vi "_fgv_attributes.vi"(6 "Attributes (empty)":T1[](array[typedef]) {"Flags" format="%08b"; "Access" items=["Read Only", "Write Only", "Read/Write"]; "Data Type" items=["Integer 32", "Double", "String", "Boolean", "None", "Integer 64", "RawString"]}, 7 "Operation":T5=enum."Get Attribute", 8 "error in":errorcluster caption="error in (no error)", 10 "Attribute ID in":string, 11 "VISA resource name":refnum<visa-resource-name>) -> (0 "error out":errorcluster, 1 "Count Out":i32, 2 "Attribute out":T2={"Identifier"="", "Descriptive Name"="", "Data Type"=enum."Integer 32", "Command"="", "Access"=enum."Read/Write", "Range Table"="", "Read Callback"="", "Write Callback"="", "Supported Models"="", "Instrument Options"="", "Index"=0, "OPC Wait"=FALSE, "No Status Check"=FALSE, "Cache Only"=FALSE}, 3 "VISA resource name out":refnum<visa-resource-name>)   [LabVIEW 2022 SP3, in "hmp4000_rsidr_core.lvlib"]
uses:
  hmp4000_rsidr_core.lvlib
  _type_Operation_Fgv_Attributes.ctl
  type_Attribute.ctl
  type_Attribute_Data_Type.ctl
  type_ReadWriteAccess.ctl
  type_Input_Format_Attribute.ctl
  type_Error_Codes.ctl
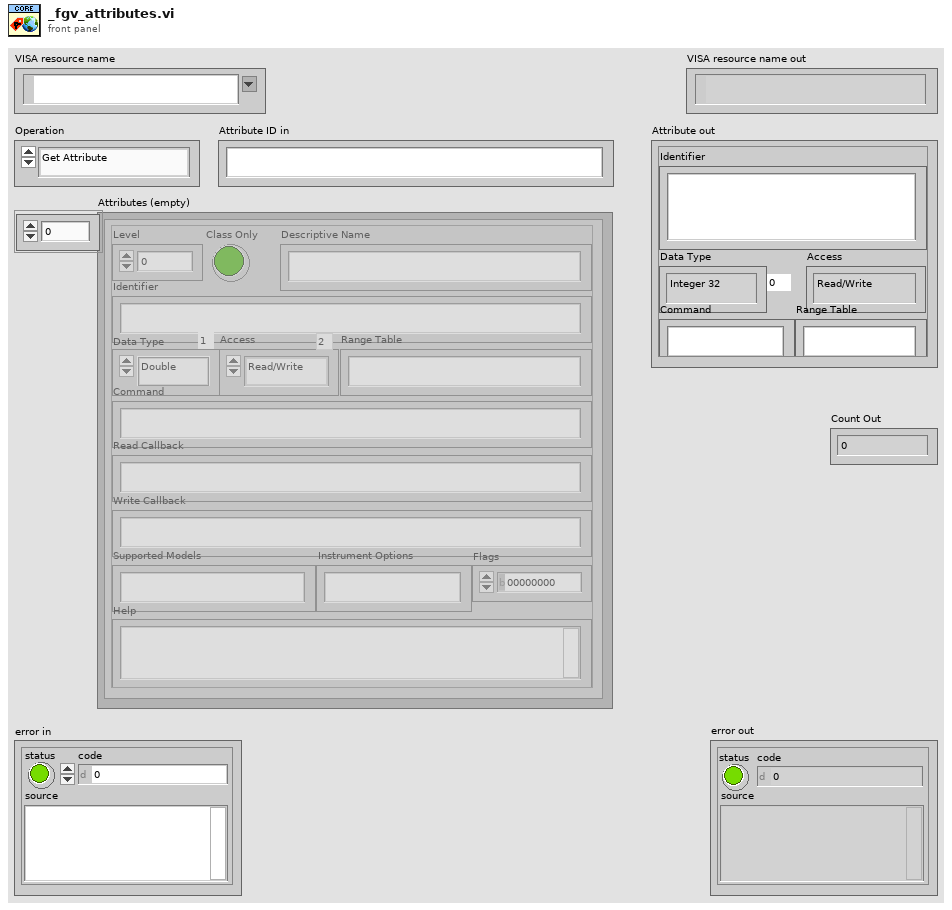
[diagram p1: front panel]
types:
  T1 = typedef "hmp4000_rsidr_core.lvlib/type_Input_Format_Attribute.ctl" = cluster{"Level":i32, "Class Only":bool, "Identifier":string, "Descriptive Name":string, "Data Type":u16, "Command":string, "Access":u16, "Range Table":string, "Read Callback":string, "Write Callback":string, "Supported Models":string, "Instrument Options":string, "Flags":i32, "Help":string}
  T2 = typedef "hmp4000_rsidr_core.lvlib/type_Attribute.ctl" = cluster{"Identifier":string, "Descriptive Name":string, "Data Type":T3, "Command":string, "Access":T4, "Range Table":string, "Read Callback":string, "Write Callback":string, "Supported Models":string, "Instrument Options":string, "Index":i32, "OPC Wait":bool, "No Status Check":bool, "Cache Only":bool}
  T3 = typedef "hmp4000_rsidr_core.lvlib/type_Attribute_Data_Type.ctl" = enum16{"Integer 32", "Double", "String", "Boolean", "None", "Integer 64", "RawString"}
  T4 = typedef "hmp4000_rsidr_core.lvlib/type_ReadWriteAccess.ctl" = enum16{"Read Only", "Write Only", "Read/Write"}
  T5 = typedef "hmp4000_rsidr_core.lvlib/_type_Operation_Fgv_Attributes.ctl" = enum16{"Initialize", "Get Attribute"}
  T6 = typedef "hmp4000_rsidr_core.lvlib/type_Error_Codes.ctl" = enum16{"No_error", "VISA_err_ResourceNotFound", "VISA_err_Timeout", "VISA_warn_MoreDataAvailable", "RS_err_MissingCallback", "RS_err_InvalidAttribute", "RS_err_InvalidValue", "RS_err_UnknownResource", "RS_err_AlreadyInitialized", "RS_err_InstrumentStatus", "RS_err_BadRepCapName", "RS_err_TypesMismatch", "RS_err_ValueNotSupported", "RS_err_InvalidRngTable", "RS_err_IDqueryFail", "RS_err_UnexpResponse", "VISA_warn_ConfigNotLoaded", "RS_err_AttributeNotReadable", "RS_err_AttributeNotWritable", "RS_err_InstrumentType", "RS_err_InstrumentOption", "VISA_err_InvalidSize", "RS_err_ReliabilityIndicator", "VISA_warn_UnknownStatus", "VISA_warn_TermCharRead", "VISA_err_IO_error", "RS_err_FunctionNotSupported", "VISA_warn_QueueEmpty"}
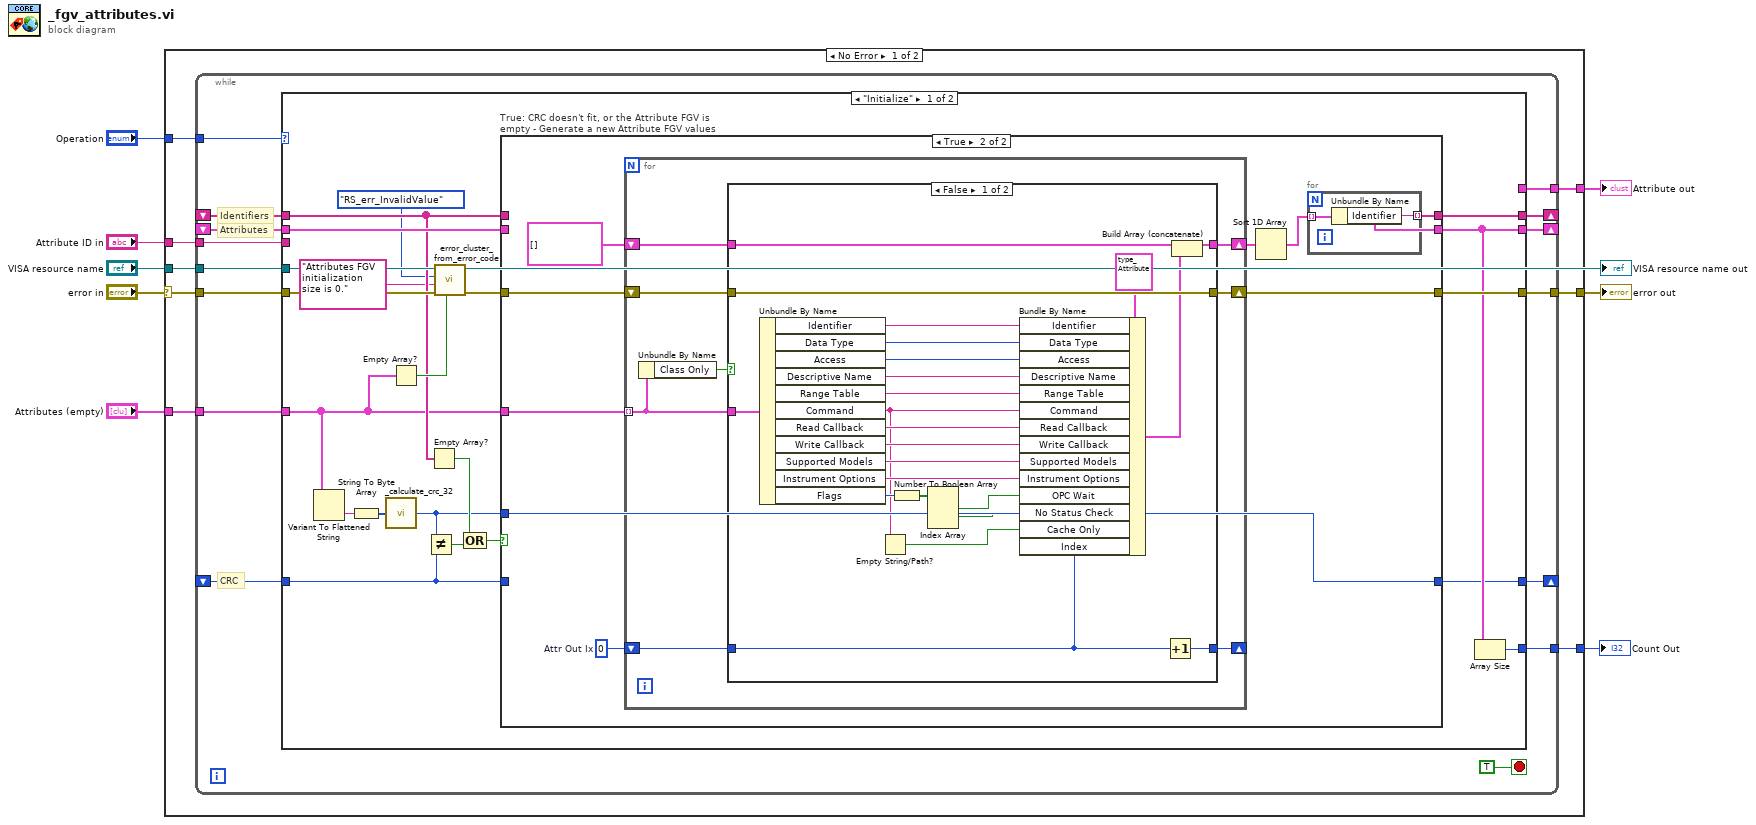
[diagram p0: block diagram]
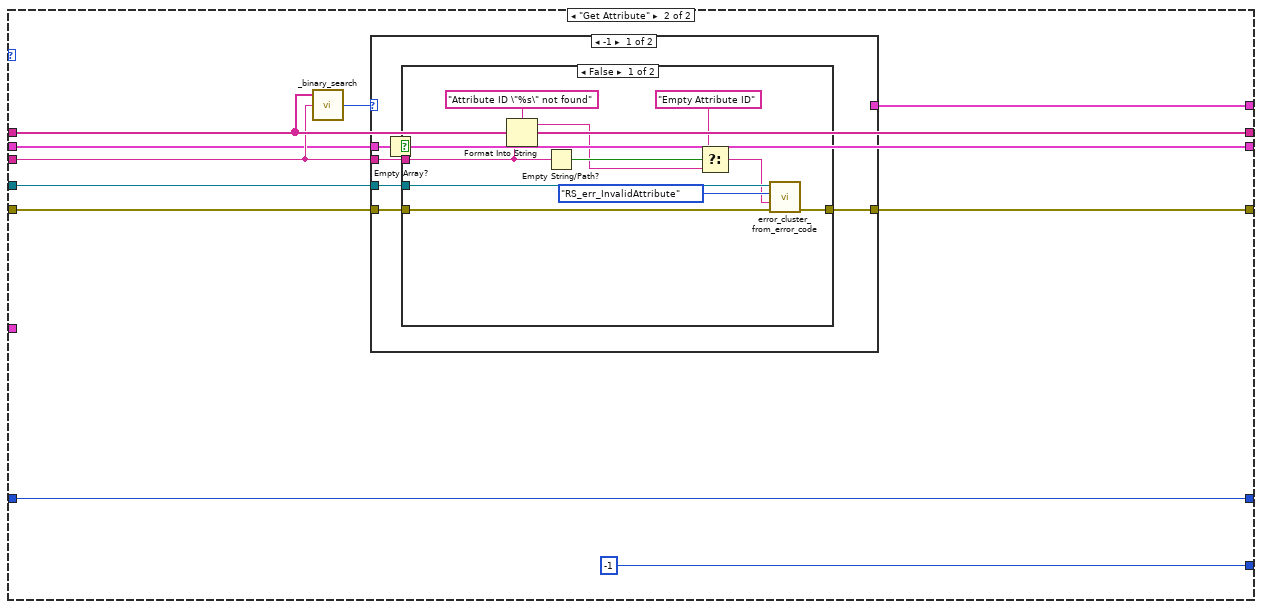
[diagram p4: hidden frame]
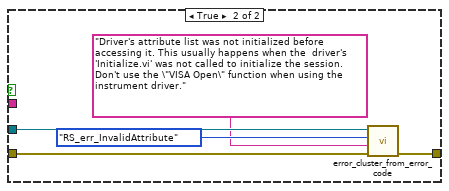
[diagram p5: hidden frame]
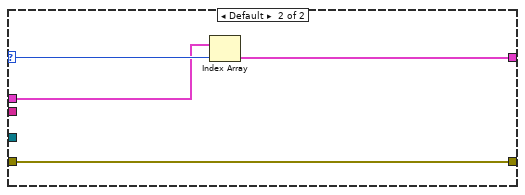
[diagram p6: hidden frame]
diagram:
  n1 = case shown="No Error" "error in" {
    selector: "error in" -> [w10 w137]
    tunnel: "Operation" -> [w16 _]
    tunnel: [w15 w137] -> w2
    tunnel: "Attribute ID in" -> [w14 _]
    tunnel: [w13 _] -> w6
    tunnel: "Attributes (empty)" -> [w12 _]
    tunnel: [w11 _] -> w4
    tunnel: "VISA resource name" -> [w9 _]
    frame No Error {
      n2 = while {
        tunnel: w16 -> [w31]
        tunnel: [w30] -> w15
        tunnel: w14 -> [w29]
        tunnel: [w28] -> w13
        tunnel: w12 -> [w27]
        tunnel: [w26] -> w11
        tunnel: w10 -> [w25]
        shift-right: [w23] -> _
        shift-left: _ -> [w22]
        shift-right: [w20] -> _
        shift-left: _ -> [w21]
        shift-right: [w18] -> _
        shift-left: _ -> [w19]
        tunnel: w9 -> [w17]
        stop <- TRUE stop-if-true
        # "Attributes"
        # "CRC"
        # "Identifiers"
        n3 = case shown="\"Initialize\"" w31 {
          tunnel: [w52 w111] -> w30
          tunnel: w29 -> [_ w106]
          tunnel: [_ w105] -> w28
          tunnel: w27 -> [w33 _]
          tunnel: [w47 -1 ("dimension size")] -> w26
          tunnel: w25 -> [w51 w108]
          tunnel: [w48 w104] -> w23
          tunnel: w22 -> [w46 w104]
          tunnel: w21 -> [w42 w109]
          tunnel: [w49 w109] -> w20
          tunnel: w19 -> [w38 w103]
          tunnel: [w36 w103] -> w18
          tunnel: w17 -> [w35 w102]
          frame "Initialize" {
            n4 = Variant To Flattened String(Variant=w33) -> (data string=w45:string)  [unwired: 1 out]
            n5 = String To Byte Array(string=w45) -> (unsigned byte array=w44:u8[])
            n6 = call "_calculate_crc_32.vi"("Data in"=w44) -> ("CRC_32"=w37:u32)  [unwired: 4 in]
            n7 = Empty Array?(array=w33) -> (empty?=w43:bool)
            n8 = Not Equal?(x=w37, y=w38) -> (x != y?=w41:bool)
            n9 = Empty Array?(array=w42) -> (empty?=w40:bool)
            n10 = call "error_cluster_from_error_code.vi"("Error Creation Enabled (True)"=w43, "error in"=w51, "Error Message (\"\")"="Attributes FGV initialization size is 0.", "Error Enum in"=type_Error_Codes."RS_err_InvalidValue", "VISA resource name"=w35) -> ("error out"=w50:errorcluster)  [unwired: 5 in, 1 out]
            n11 = Compound Arithmetic op=OR(w40, w41) -> (w39:bool)
            n12 = case "True: CRC doesn't fit, or the Attribute FGV is empty - Generate a new Attribute FGV values" shown="True" w39 {
              tunnel: [w54 w64] -> w52
              tunnel: w50 -> [w54 w62]
              tunnel: w33 -> [_ w61]
              tunnel: [w56 w60] -> w49
              tunnel: [w55 w59] -> w48
              tunnel: w42 -> [w56 _]
              tunnel: w46 -> [w55 _]
              tunnel: w38 -> [w53 _]
              tunnel: w37 -> [_ w57]
              tunnel: [w53 w57] -> w36
              frame False {
              }
              frame True {
                w65 = 0  # Attr Out Ix
                n13 = for {
                  tunnel: w61 -> [w68] mode=indexing
                  shift-right: [w73] -> _
                  shift-left: w65 -> [w74]
                  shift-right: [w71] -> w64
                  shift-left: w62 -> [w72]
                  shift-right: [w69] -> w63
                  shift-left: T2[] [] -> [w70]
                  n14 = Unbundle By Name(w68) -> ("Class Only"=w75:bool)
                  n15 = case shown="False" w75 {
                    tunnel: w68 -> [w88 _]
                    tunnel: w74 -> [w85 w101]
                    tunnel: [w98 w101] -> w73
                    tunnel: w72 -> [w91 w100]
                    tunnel: [w91 w100] -> w71
                    tunnel: w70 -> [w90 w99]
                    tunnel: [w89 w99] -> w69
                    frame False {
                      n16 = Unbundle By Name(w88) -> ("Identifier"=w86:string, "Data Type"=w97:u16, "Access"=w96:u16, "Descriptive Name"=w95:string, "Range Table"=w92:string, "Command"=w77:string, "Read Callback"=w94:string, "Write Callback"=w93:string, "Supported Models"=w80:string, "Instrument Options"=w79:string, "Flags"=w84:i32)
                      n17 = Empty String/Path?(string/path=w77) -> (empty?=w76:bool)
                      n18 = Number To Boolean Array(number=w84) -> (Boolean array=w83:bool[])
                      n19 = Index Array(array=w83) -> (element #1=w82:bool, element #2=w81:bool)  [unwired: 3 in, 1 out]
                      n20 = Bundle By Name(cluster=T2 {"Identifier"="", "Descriptive Name"="", "Data Type"=enum."Integer 32", "Command"="", "Access"=enum."Read/Write", "Range Table"="", "Read Callback"="", "Write Callback"="", "Supported Models"="", "Instrument Options"="", "Index"=0, "OPC Wait"=FALSE, "No Status Check"=FALSE, "Cache Only"=FALSE} ("Attribute"), "Identifier"=w86, "Data Type"=w97, "Access"=w96, "Descriptive Name"=w95, "Range Table"=w92, "Command"=w77, "Read Callback"=w94, "Write Callback"=w93, "Supported Models"=w80, "Instrument Options"=w79, "OPC Wait"=w82, "No Status Check"=w81, "Cache Only"=w76, "Index"=w85) -> (w87:T2)
                      n21 = Increment(x=w85) -> (x+1=w98:i32)
                      n22 = Build Array (concatenate)(w90, w87) -> (w89:T2[])
                    }
                    frame True {
                    }
                  }
                }
                n23 = Sort 1D Array(array=w63) -> (sorted array=w59:T2[])
                n24 = for {
                  tunnel: w59 -> [w67] mode=indexing
                  tunnel: [w66] -> w60 mode=indexing
                  n25 = Unbundle By Name(w67) -> ("Identifier"=w66:string)
                }
              }
            }
            n26 = Array Size(array=w48) -> (size(s)=w47:i32)
          }
          frame "Get Attribute" {
            n27 = call "_binary_search.vi"("String to search"=w106, "Strings in"=w109) -> ("Index out"=w107:i32)  [unwired: 3 in]
            n28 = case shown="-1" w107 {
              selector: w107 -> [_ w135]
              tunnel: [w117 w136] -> w111
              tunnel: w108 -> [w116 w136]
              tunnel: w106 -> [w115 _]
              tunnel: [_ w134] -> w105
              tunnel: w104 -> [w113 w133]
              tunnel: w102 -> [w114 _]
              frame -1 {
                n29 = Empty Array?(array=w113) -> (empty?=w112:bool)
                n30 = case shown="False" w112 {
                  tunnel: [w127 w132] -> w117
                  tunnel: w116 -> [w126 w131]
                  tunnel: w115 -> [w121 _]
                  tunnel: w114 -> [w123 w129]
                  frame False {
                    n31 = Format Into String(format string="Attribute ID \"%s\" not found", w121) -> (resulting string=w120:string)  [unwired: 2 in, 1 out]
                    n32 = Empty String/Path?(string/path=w121) -> (empty?=w122:bool)
                    n33 = Select(t="Empty Attribute ID", s=w122, f=w120) -> (s? t:f=w118:string)
                    n34 = call "error_cluster_from_error_code.vi"("error in"=w126, "Error Message (\"\")"=w118, "Error Enum in"=type_Error_Codes."RS_err_InvalidAttribute", "VISA resource name"=w123) -> ("error out"=w127:errorcluster)  [unwired: 6 in, 1 out]
                  }
                  frame True {
                    n35 = call "error_cluster_from_error_code.vi"("error in"=w131, "Error Message (\"\")"="Driver's attribute list was not initialized before accessing it. This usually happens when the  driver's 'Initialize.vi' was not called to initialize the session. Don't use the \"VISA Open\" function when using the instrument driver." ("format string"), "Error Enum in"=type_Error_Codes."RS_err_InvalidAttribute", "VISA resource name"=w129) -> ("error out"=w132:errorcluster)  [unwired: 6 in, 1 out]
                  }
                }
              }
              frame Default {
                n36 = Index Array(array=w133, index=w135) -> (element=w134:T2)
              }
            }
          }
        }
      }
    }
    frame Error {
    }
  }
  "error out" <- w2
  "Attribute out" <- w6
  "Count Out" <- w4
  "VISA resource name out" <- "VISA resource name"
